vi "Camera Process.vi"   [LabVIEW 2013]
uses:
  Camera Global.vi
types:
  T1 = cluster{"Manual X Angle":dbl, "Manual Y Angle ":dbl, "Set X Angle":dbl, "Set Y Angle ":dbl, "Wanted X Angle":dbl, "Wanted Y Angle  ":dbl}
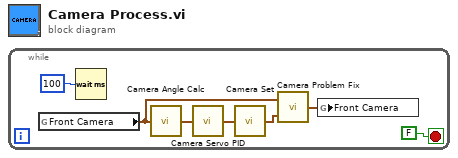
[diagram p0: block diagram]
diagram:
  n1 = while {
    stop <- FALSE stop-if-true
    n2 = global read "Camera Global.vi" "Front Camera"() -> (w2:T1)
    n3 = Wait (ms)(milliseconds to wait=u32 100) -> ()  [unwired: 1 out]
    n4 = call "Camera Angle Calc.vi"("Front Camera In"=w2) -> ("Front Camera Out"=w5:T1)
    n5 = call "Camera Servo PID.vi"("Front Camera In"=w5) -> ("Front Camera Out"=w4:T1)
    n6 = call "Camera Set.vi"("Front Camera In"=w4) -> ("Front Camera Out"=w3:T1)
    n7 = call "Camera Problem Fix.vi"("Front Camera Modified"=w3, "Front Camera Original"=w2) -> ("Front Camera Fixed"=w1:T1)
    n8 = global write "Camera Global.vi" "Front Camera"(w1) -> ()
  }
